vi "BinChecker.vi"(10 "Lower Bins":dbl[](array[numeric]), 11 "Upper Bins":dbl[](array[numeric])) -> (3 "Boolean":bool)   [LabVIEW 2012, in "Histogram Custom Device.lvlib"]
uses:
  Histogram Custom Device.lvlib
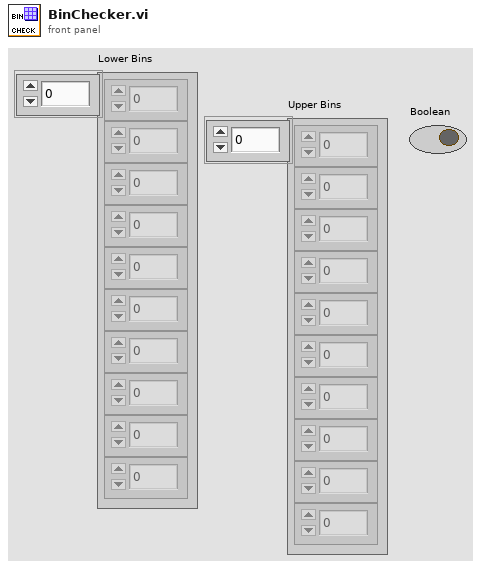
[diagram p1: front panel]
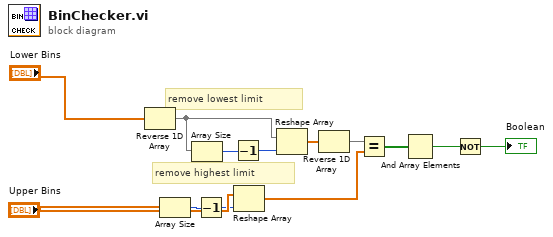
[diagram p0: block diagram]
diagram:
  # "remove highest limit"
  # "remove lowest limit"
  n1 = Reverse 1D Array(array="Lower Bins") -> (reversed array=w1:dbl[])
  n2 = Array Size(array="Upper Bins") -> (size(s)=w5:i32)
  n3 = Array Size(array=w1) -> (size(s)=w2:i32)
  n4 = Decrement(x=w5) -> (x-1=w6:i32)
  n5 = Decrement(x=w2) -> (x-1=w3:i32)
  n6 = Reshape Array("Upper Bins", w6) -> (w10:dbl[])
  n7 = Reshape Array(w1, w3) -> (w4:dbl[])
  n8 = Reverse 1D Array(array=w4) -> (reversed array=w9:dbl[])
  n9 = Equal?(x=w9, y=w10) -> (x = y?=w11:bool[])
  n10 = And Array Elements(Boolean array=w11) -> (logical AND=w12:bool)
  n11 = Not(x=w12) -> (.not. x?=→"Boolean":bool)
